vi "controller.vi"(3 "Number C":dbl, 4 "Number B":dbl, 5 "Number A":dbl) -> (0 "RESULT B":dbl, 1 "RESULT C":dbl, 2 "RESULT A":dbl)   [LabVIEW 2021]
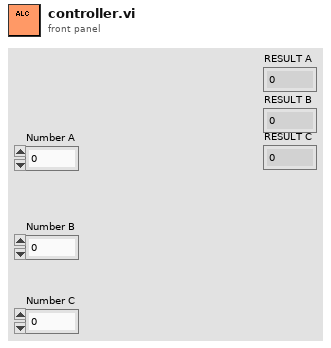
[diagram p1: front panel]
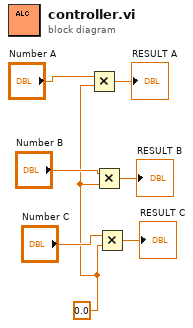
[diagram p0: block diagram]
diagram:
  w1 = 0.0 ("Number C")
  n1 = Multiply(x="Number A", y=w1) -> (x*y=→"RESULT A":dbl)
  n2 = Multiply(x="Number B", y=w1) -> (x*y=→"RESULT B":dbl)
  n3 = Multiply(x="Number C", y=w1) -> (x*y=→"RESULT C":dbl)
